vi "Database.WriteStationValues.vi"(8 "error in":errorcluster, 10 "FileName":string, 11 "Data in":T3 {"Variant"."TS"."TV"."minimum" format="%#.3f"; "Variant"."TS"."TV"."maximum" format="%#.3f"; "Variant"."TS"."TP"."value" format="%#.3f"}) -> (0 "error out":errorcluster, 3 "Data out":T3 {"Variant"."TS"."TV"."minimum" format="%#.3f"; "Variant"."TS"."TV"."maximum" format="%#.3f"; "Variant"."TS"."TP"."value" format="%#.3f"})   [LabVIEW 2016]
doc: "Write test results (measurement values) to proda database\n\nWabco 2017 All right reserved\nAuthor: maciej.szupienko@wabco-auto.com"
uses:
  Database.Main.Data.ctl
  Database.Main.Data.Status.ctl
  Database.Main.Data.Sets.ctl
  Database.Main.Data.Results.ctl
  Sequence/Sequence.Step.Status.ctl
  ProdaNG/Controls/ProdaNG.Identification.ctl
  ProdaNG/Controls/ProdaNG.ProcessResult.ctl
  ProdaNG/Controls/ProdaNG.ProcessStepResult.ctl
  ProdaNG/Controls/ProdaNG.TestStepResult.ctl
  ProdaNG/Controls/ProdaNG.TestValueResult.ctl
  Database.Main.Data.Variant.ctl
  ProdaNG/Controls/ProdaNG.ProcessStepParam.ctl
  ProdaNG/Controls/ProdaNG.TestStep.ctl
  ProdaNG/Controls/ProdaNG.TestStepParam.ctl
  ProdaNG/Controls/ProdaNG.TestValue.ctl
  tools/Translator/Translator.Message.ctl
  tools/EventLog/EventLog.EventSource.ctl
  Global/ApplicationGlobal.vi
  tools/EventLog/EventLog.New(single).vi
panel:
  out "Array 3":string[](array[string])
  out "Array 2":u64[][](array[numeric])
  out "Array":T2(array[cluster])
  out "Prod saved":bool
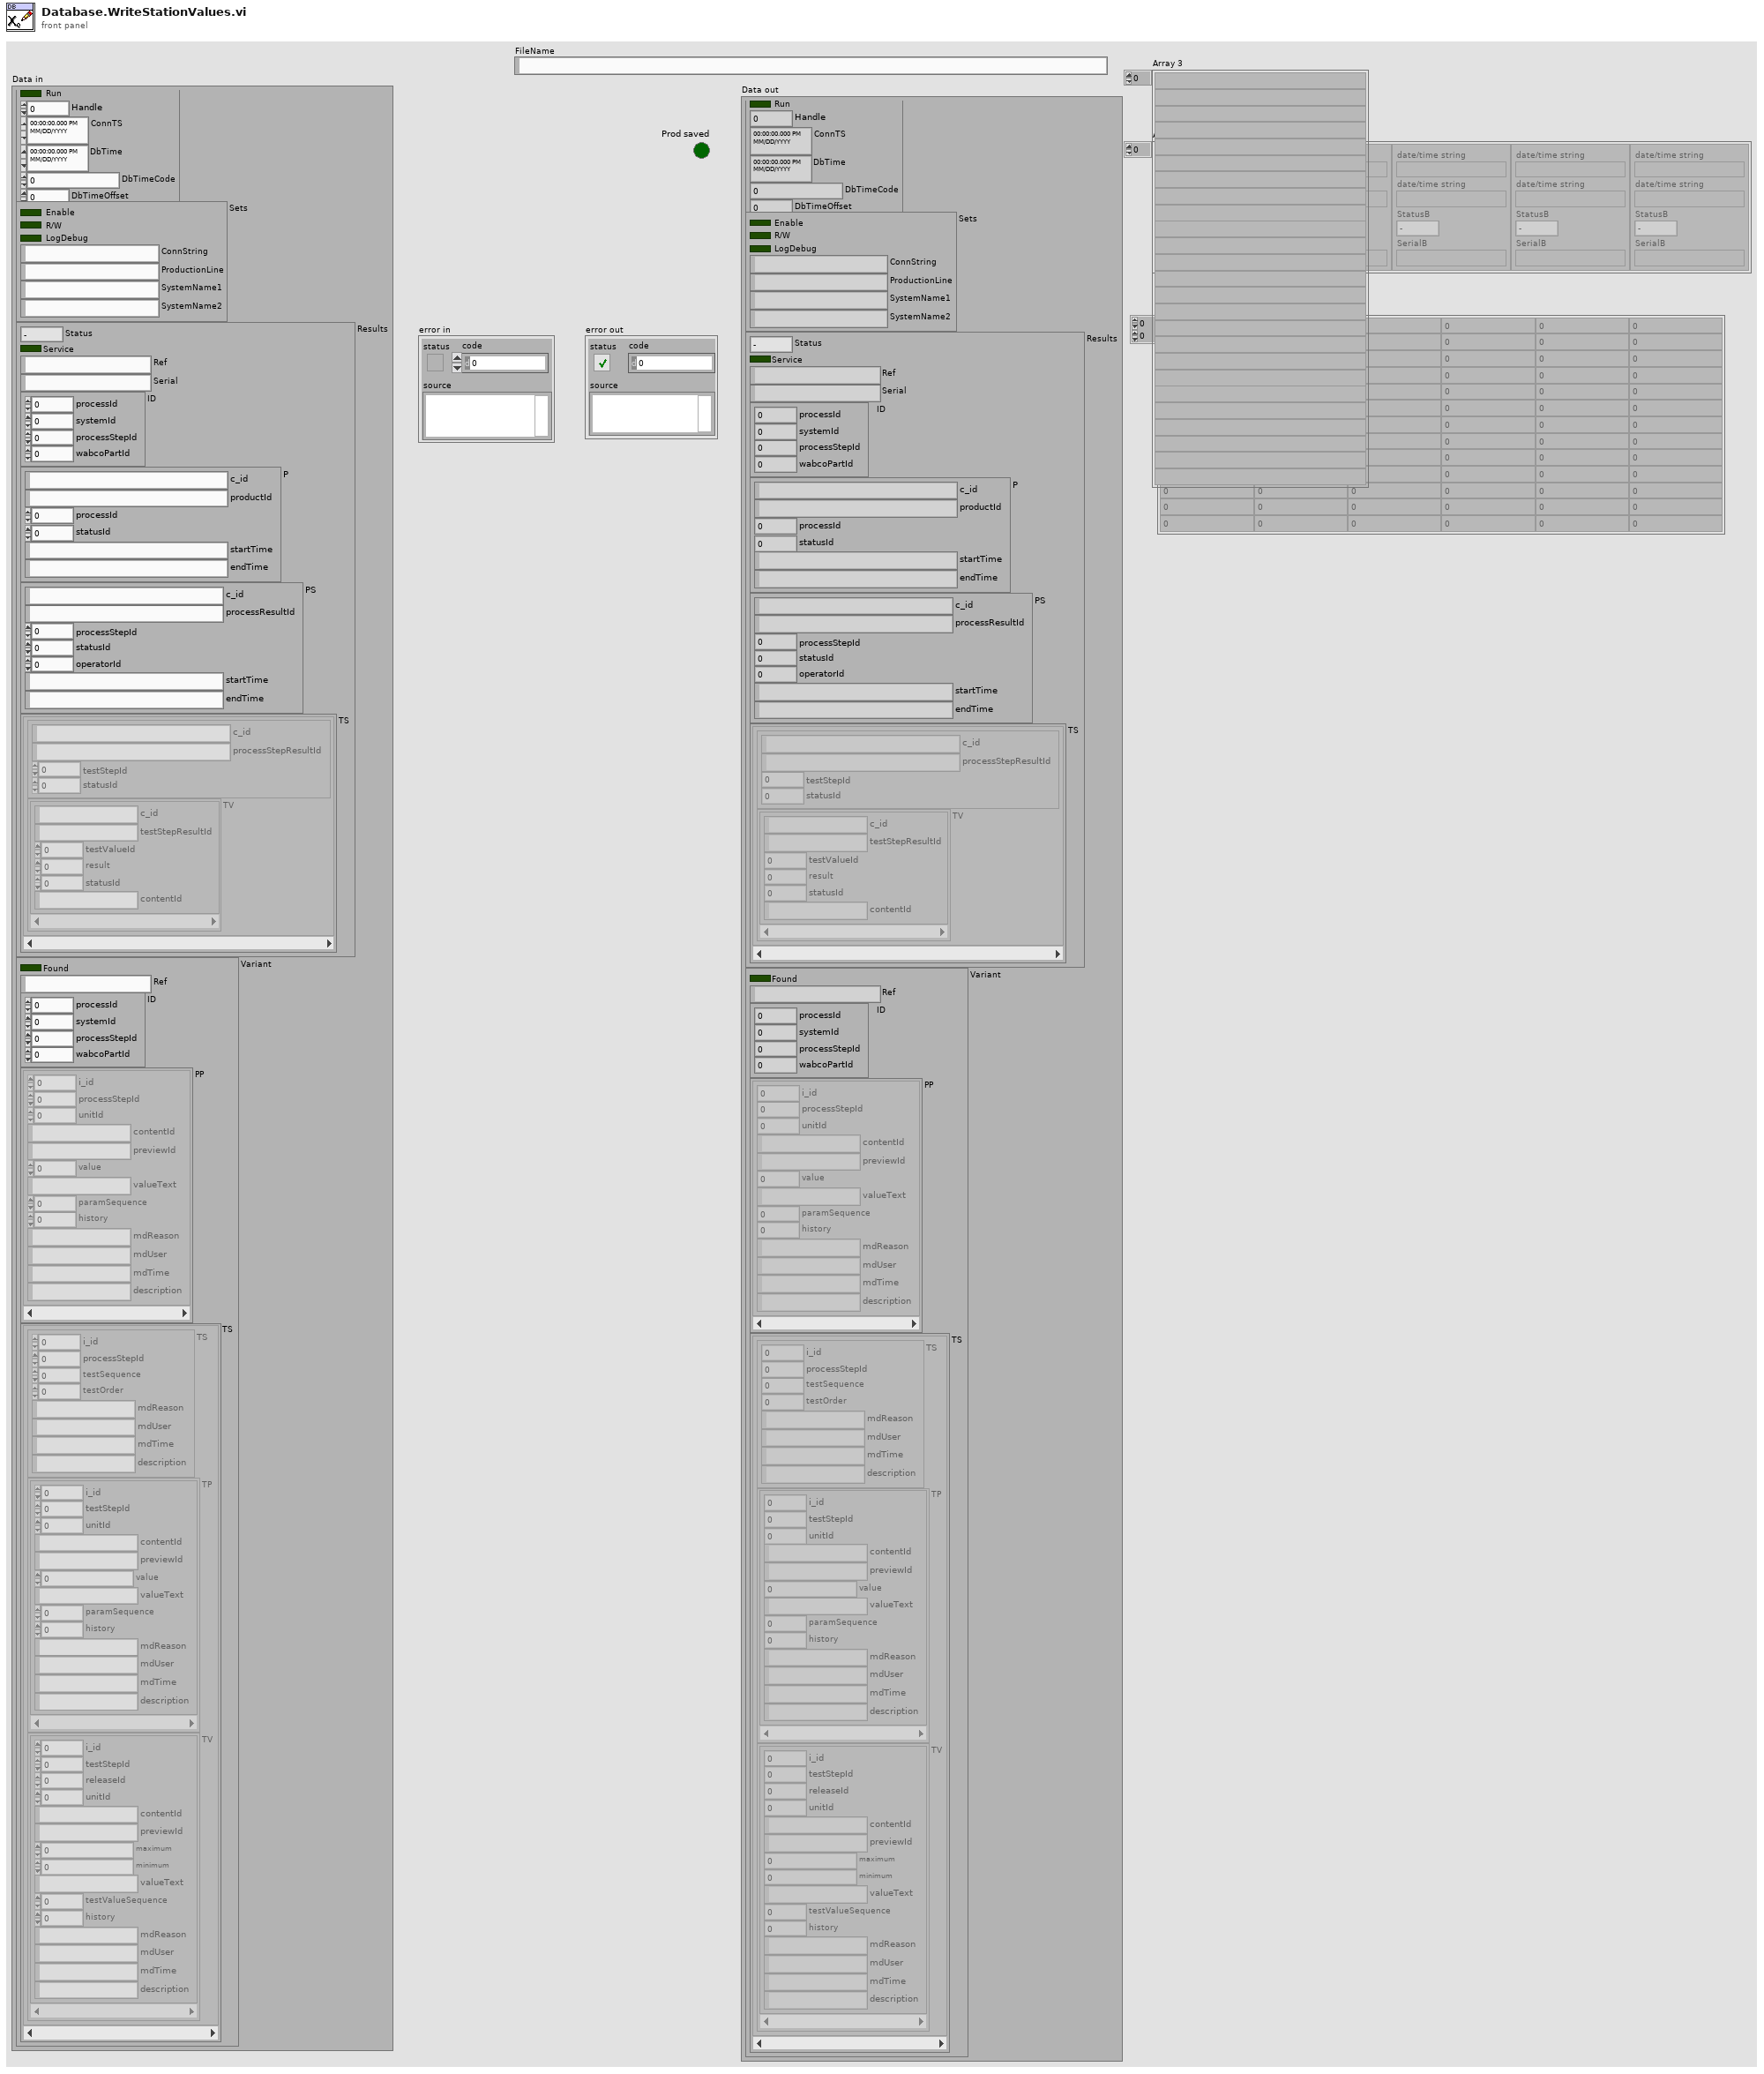
[diagram p1: front panel]
types:
  T1 = typedef "Sequence.Step.Status.ctl" = enum16{"-", "Pending", "Running", "Skipped", "Passed", "Failed", "Done", "Error", "Aborted", "Stopped"}
  T2 = cluster{"date/time string":string, "date/time string":string, "StatusB":T1, "SerialB":string}[]
  T3 = typedef "Database.Main.Data.ctl" = cluster{"Status":T4, "Sets":T5, "Results":T6, "Variant":T12}
  T4 = typedef "Database.Main.Data.Status.ctl" = cluster{"Run":bool, "Handle":i32, "ConnTS":timestamp, "DbTime":timestamp, "DbTimeCode":dbl, "DbTimeOffset":dbl}
  T5 = typedef "Database.Main.Data.Sets.ctl" = cluster{"Enable":bool, "R/W":bool, "LogDebug":bool, "ConnString":string, "ProductionLine":string, "SystemName1":string, "SystemName2":string}
  T6 = typedef "Database.Main.Data.Results.ctl" = cluster{"Status":T1, "Service":bool, "Ref":string, "Serial":string, "ID":T7, "P":T8, "PS":T9, "TS":cluster{"TS":T10, "TV":T11[]}[]}
  T7 = typedef "ProdaNG.Identification.ctl" = cluster{"processId":i32, "systemId":i32, "processStepId":i32, "wabcoPartId":i32}
  T8 = typedef "ProdaNG.ProcessResult.ctl" = cluster{"c_id":string, "productId":string, "processId":i32, "statusId":i32, "startTime":string, "endTime":string}
  T9 = typedef "ProdaNG.ProcessStepResult.ctl" = cluster{"c_id":string, "processResultId":string, "processStepId":i32, "statusId":i32, "operatorId":i32, "startTime":string, "endTime":string}
  T10 = typedef "ProdaNG.TestStepResult.ctl" = cluster{"c_id":string, "processStepResultId":string, "testStepId":i32, "statusId":i32}
  T11 = typedef "ProdaNG.TestValueResult.ctl" = cluster{"c_id":string, "testStepResultId":string, "testValueId":i32, "result":dbl, "statusId":i32, "contentId":string}
  T12 = typedef "Database.Main.Data.Variant.ctl" = cluster{"Found":bool, "Ref":string, "ID":T7, "PP":T13[], "TS":cluster{"TS":T14, "TP":T15[], "TV":T16[]}[]}
  T13 = typedef "ProdaNG.ProcessStepParam.ctl" = cluster{"i_id":i32, "processStepId":i32, "unitId":i32, "contentId":string, "previewId":string, "value":dbl, "valueText":string, "paramSequence":i32, "history":i32, "mdReason":string, "mdUser":string, "mdTime":string, "description":string}
  T14 = typedef "ProdaNG.TestStep.ctl" = cluster{"i_id":i32, "processStepId":i32, "testSequence":i32, "testOrder":i32, "mdReason":string, "mdUser":string, "mdTime":string, "description":string}
  T15 = typedef "ProdaNG.TestStepParam.ctl" = cluster{"i_id":i32, "testStepId":i32, "unitId":i32, "contentId":string, "previewId":string, "value":dbl, "valueText":string, "paramSequence":i32, "history":i32, "mdReason":string, "mdUser":string, "mdTime":string, "description":string}
  T16 = typedef "ProdaNG.TestValue.ctl" = cluster{"i_id":i32, "testStepId":i32, "releaseId":i32, "unitId":i32, "contentId":string, "previewId":string, "maximum":dbl, "minimum":dbl, "valueText":string, "testValueSequence":i32, "history":i32, "mdReason":string, "mdUser":string, "mdTime":string, "description":string}
  T17 = typedef "EventLog.EventSource.ctl" = enum16{"All", "Gui", "Ref", "File", "Arch", "Seq", "CPX", "DB", "Laser", "Scan.P", "Scan.O"}
  T18 = typedef "Translator.Message.ctl" = enum16{"-", "Event confirmed", "Log out", "Log in", "Shutdown", "Cancel", "Start", "Begin time", "End time", "Duration", "Service Mode", "Ignore Results", "Serial Format", "On", "Off", "OK", "NOK", "NOK %s", "Home", "Work", "Close", "Open", "In progress...", "Missing", "Empty", "Hardware failure", "Initial", "Default", "Total", "Out of range", "Free disk space is below 1GB - contact technician", "Error %d >> %s", "Error %d >> %s >> %s", "Msg %d >> %s", "Laser msg %d %s", "Laser cmd error %s %d", "Laser cmd failed %s", "Laser cmd warning %s", "Laser disconnected", "Laser status %s", "Laser already started", "Laser job unkonwn %s", "Laser job missing %s", "Laser job select failure %s", "Unable to start laser printing (%s)", "Unable to stop laser printing (%s)", "Laser marking aborted", "Laser marking timeout", "Unable to reset Laser Interlock (%s)", "Unable to trigger Laser. Laser not ready (%s)", "Laser job '%s' coordinates not configured", "Starting %s", "Quitting %s", "Configured", "Initializing", "Quitting", "Loading", "Loaded %d results", "Loaded %d events", "Running", "Stopped", "Summary", "Laser", "Do you want to continue?", "Do you want to delete the configuration?", "The configuration is being used by an order. Unable to delete!", "Press confirm button", "Station is not based. Do you want to exit?", "Station requires changeover. Do you want to run the test?", "Test options are not set as default. Do you want to continue?", "Formatting of WabcoNo is disabled. Do you want to continue?", "Product not detected. Do you want to continue?", "Product scan failed. Do you want to continue?", "Calibration", "Log out?", "System", "All", "IDLE", "Translating...%s", "Not found", "Alarm %s", "Run", "Skip", "Abort", "Repeat", "Please wait...", "Database disconnected", "Database disconnected - changeover disabled!", "Login to database successful", "Login to database failed: %d; %s", "Unable to check the product status of reference %d - database disconnected", "Unable to set the product status of reference %d - database disconnected", "Variant file backup %s", "Read variant (%s)", "Result", "Station armed!", "Station requires changeover!", "Select reference number...", "EMERGENCY BUTTON - press Control button", "EMERGENCY DOOR - press Control button", "Resetting Emergency...", "Unable to reset safety circuit - Emergency Button pressed", "Unable to reset safety circuit - Emergency Side Door open", "Station not based", "Station based", "Station not empty", "Station basing...", "No order", "Press Start to begin new order", "Scanning new order", "Order NOK. Correct or scan again", "Order OK. Press Accept", "Order ready", "Revolver incorrect", "Fork incorrect", "Revolver missing", "Revolver empty", "Container missing", "Offline results", "Offline statistics", "Updating statistics %.1f %%", "DMC Configurator", "Door open", "Close the front door", "Press start button", "Done. Open the front door", "Running...", "Running...%.1f %%", "Pause %s", "Pause %s. NOK container missing", "Pause %s. OK container missing", "Pause %s. Revolver empty", "Pause %s. Revolver missing", "Pause %s. Revolver incorrect", "Pause %s. Fork missing", "Pause %s. Fork incorrect", "Pause %s. Too many failures", "Pause %s. Unloading failure", "Pause %s. One slot is not working", "Pause %s. Part order is done. Empty OK container", "Pause %s. Unable to move product to slot", "Pause %s. Unable to move back product pusher", "Pause %s. Unable to lift product", "Pause %s. Unable to move back product lifter", "Pause %s. Unable to move product arm to Work", "Pause %s. Unable to move product arm to NOK", "Pause %s. Unable to move product arm to OK", "Pause %s. Unable to unsuck the NOK product", "Pause %s. Unable to drop the NOK product", "Pause %s. Product OK missing", "Pause %s. Unable to unsuck the OK product", "Pause %s. Unable to drop the OK product", "Stopping...", "File '%s' is missing", "File '%s' is broken", "File '%s' is running", "Log file started (%s)", "Log file ended (%s)", "Log file stopped (%s)", "Log file ignored (%s)", "Log file exported (%s)", "Log file export failed (%s)", "Wrong serial number in log file", "Wrong reference number in log file", "Test steps are missing", "%s = %.3f", "Process param '%s' not found in DB", "Process param '%s' wrong order", "Process param '%s' value %.3f out of limits (%.3f; %.3f)", "Step%d param '%s' not found in DB", "Step%d param '%s' wrong order", "Step%d param '%s' value %.3f out of limits (%.3f; %.3f)", "Step%d EV '%s' not found in DB", "Step%d EV '%s' wrong order", "\"%s\" not found in DB", "\"%s\" wrong order", "\"%s\" value %.3f out of limits (%.3f; %.3f)", "\"%s\" not found in software", "Process init (%s)", "Process started", "Process restarted", "Process run", "Process done", "Process done - remove OK container", "Process aborted", "Process aborted at work", "Process aborted at home", "Process error", "Process error at home", "Process error at work", "Process close", "Process pause", "Process continue", "Process door open", "Process door close", "Process pause at slot %s due to %s", "Select plate from the order to process", "Do you want to start the process?", "Do you want to continue the process?", "There is unfinished order. Do you want to put the new order?", "Product %s %d OK", "Product %s %d NOK", "Unable to unload the slot %s. Product missing in the slot", "Unable to unload the slot %s. Product already in the arm", "Unable to accept the product as OK. Product missing in slot %s", "Unable to accept the product as OK. Product could not drop into the container at slot %s", "Unable to accept the product as NOK. Product could not drop into the container at slot %s", "Scan failed. Error %s", "Scan failed. Scanner disconnected", "Scan failed. Wrong Wabco number %d, limit (%d,%d)", "Scan failed. Wrong serial number %d, limit (%d,%d)", "Scan failed. Wrong date %d, limit (%d,%d)", "Scan failed. Wrong product wabco number %d (expected %d)", "Scan failed. Wrong product serial number %d (expected > 0)", "Scan OK %s", "Scan failed. Unable to determine table position (%s)", "Scan failed. Timeout", "Tune failed. Scanner disconnected", "Tune failed. Timeout", "%s = %d", "%s = %d->%d", "Unable to set %s = %.2f - Air Pressure Inside off", "Unable to set digital output '%s' = %d", "Unable to activate air pressure inside - timeout", "Unable to activate air pressure inside - aborted", "Unable to switch on Air Main Valve - Air Pressure Inlet off", "Unable to switch on Air Main Valve - Door open", "Unable to switch off Air Main Valve - timeout", "Unable to switch off Air Main Valve - aborted", "Unable to rotate Table - timeout", "Unable to rotate Table - aborted", "Unable to rotate Table - Product Move not in Home position", "Unable to rotate Table - Air Pressure Inside off", "Unable to rotate Table - Product Lift A not in Home position", "Unable to rotate Table - Product Lift B not in Home position", "Unable to rotate Table - unlock before movement timeout", "Unable to rotate Table - lock after movement timeout", "Unable to move Table Lock to %s position - timeout", "Unable to move Table Lock to %s position - aborted", "Unable to move Table Lock to %s position - Air Pressure Inside off", "Unable to move Table Lock to %s position - Table not in position", "Unable to move Product Lift A to %s position - timeout", "Unable to move Product Lift B to %s position - timeout", "Unable to move Product Lift A to %s position - aborted", "Unable to move Product Lift B to %s position - aborted", "Unable to move Product Lift A to %s position - Air Pressure Inside off", "Unable to move Product Lift B to %s position - Air Pressure Inside off", "Unable to move Product Lift A to %s position - Table not locked", "Unable to move Product Lift B to %s position - Table not locked", "Unable to move Product Lift A to %s position - Product Arm not in Work position", "Unable to move Product Lift B to %s position - Product Arm not in Work position", "Unable to set Product Suction Gripper %s to %s - timeout", "Unable to set Product Suction Gripper %s to %s - aborted", "Unable to set Product Suction Gripper %s to %s - Air Pressure Inside off", "Unable to set Product Suction Gripper %s to %s - Table slot unkown", "Unable to move Product Arm to %s position - timeout", "Unable to move Product Arm to %s position - aborted", "Unable to move Product Arm to %s position - Air Pressure Inside off", "Unable to move Product Arm to %s position - Product Lift A not in Home position", "Unable to move Product Arm to %s position - Product Lift B not in Home position", "Unable to move Product to %s position - timeout", "Unable to move Product to %s position - aborted", "Unable to move Product to %s position - Air Pressure Inside off", "Unable to move Product to %s position - Table not in position"}
  T19 = typedef "Logger.File.ctl" = cluster{"Props":T20, "Data":T23[]}
  T20 = typedef "Logger.File.Properties.ctl" = cluster{"FilePath":path, "ImgFolder":string, "Ref":string, "Serial":string, "SerialFormat":T21, "Duration":dbl, "Time From":timestamp, "Time To":timestamp, "Service":bool, "IgnoreImgs":bool, "CheckDMC":bool, "Counters":T22, "Err":errorcluster}
  T21 = typedef "Sequence.Code.SerialFormat.ctl" = enum8{"", "6 dig", "7 dig"}
  T22 = typedef "Sequence.Counters.ctl" = cluster{"Expected":u16, "Done":u16, "OK":u16, "NOK":u16, "NOKlimit":u16, "Part":u16, "PartOK":u16}
  T23 = typedef "Logger.File.Serials.ctl" = cluster{"TS from":timestamp, "TS to":timestamp, "SlotID":u8, "StatusA":T1, "LaserVariablesA":string, "ScannerReadOutA":string, "ImgA":string, "CornersA":cluster{"X":i32, "Y":i32}[], "OCRIgnoredA":string, "SerialA":u8, "StatusB":T1, "LaserVariablesB":string, "ScannerReadOutB":string, "ImgB":string, "CornersB":cluster{"X":i32, "Y":i32}[], "SerialB":u8, "OCRIgnoredB":string, "CaptionA":string, "CaptionB":string}
  T24 = cluster{"date/time string":string, "date/time string":string, "StatusA":T1, "LaserVariablesA":string}
  T25 = cluster{"date/time string":string, "date/time string":string, "StatusB":T1, "LaserVariablesB":string}
  T26 = cluster{"date/time string":string, "date/time string":string, "StatusB":T1, "LaserVariablesB":string}[]
  T27 = typedef "ProdaNG.Product.ctl" = cluster{"c_id":string, "wabcoPartId":i32, "serialNumber":string, "comment":string, "individual":i32, "crProcessStepId":i32, "mdProcessStepId":i32, "crTime":string, "mdTime":string}
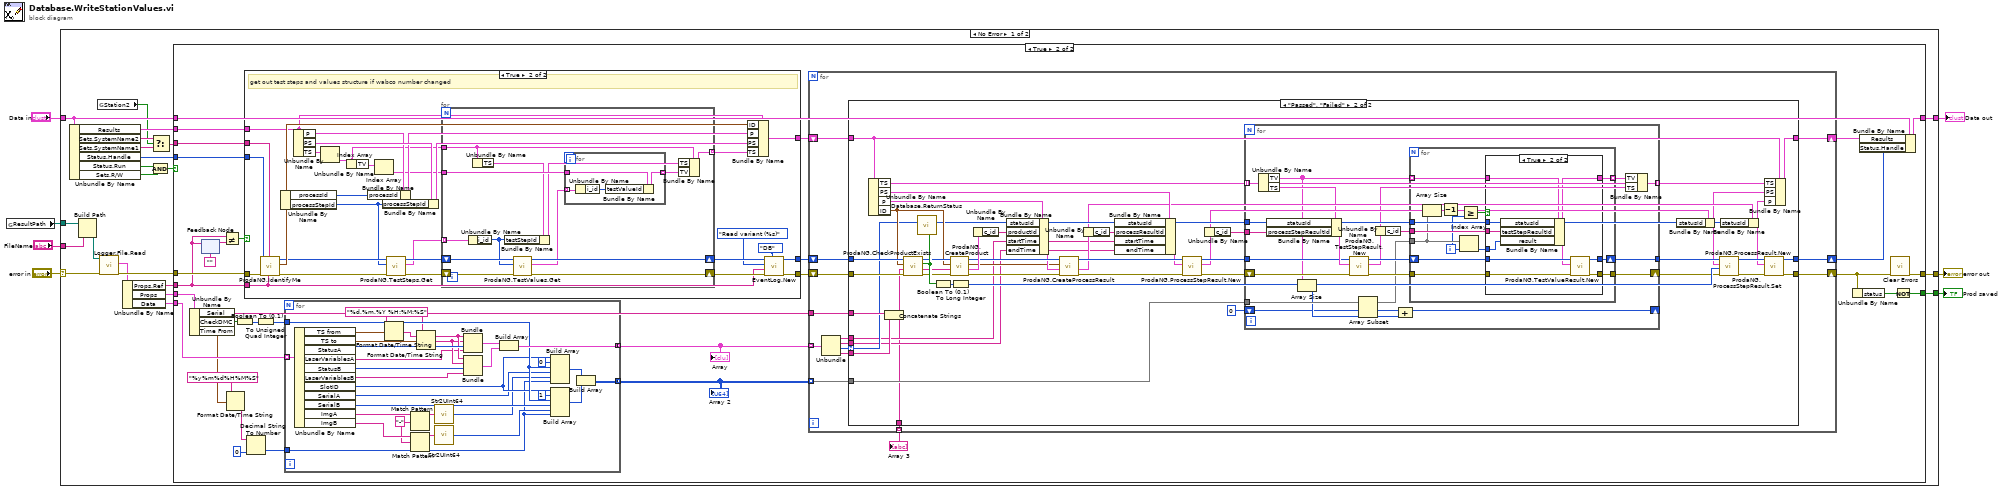
[diagram p0: block diagram]
diagram:
  n1 = global read "ApplicationGlobal.vi" "ResultPath"() -> (w2:path)
  n2 = case shown="No Error" "error in" {
    selector: "error in" -> [w13 w253]
    tunnel: [w25 w253] -> w7
    tunnel: "Data in" -> [w28 w252]
    tunnel: [w27 w252] -> w4
    tunnel: [w23 _] -> w3
    tunnel: w2 -> [w16 _]
    tunnel: "FileName" -> [w15 _]
    frame No Error {
      n3 = Unbundle By Name(w28) -> ("Results"=w26:T6, "Sets.SystemName2"=w20:string, "Sets.SystemName1"=w19:string, "Status.Handle"=w29:i32, "Status.Run"=w24:bool, "Sets.R/W"=w21:bool)
      n4 = Build Path(base path=w16, name or relative path=w15) -> (appended path=w14:path)
      n5 = global read "ApplicationGlobal.vi" "Station2"() -> (w18:bool)
      n6 = call "Logger.File.Read.vi"("error in (no error)"=w13, "file path"=w14) -> ("error out"=w12:errorcluster, "File content"=w11:T19)  [unwired: 6 in, 2 out]
      n7 = Unbundle By Name(w11) -> ("Props.Ref"=w10:string, "Props"=w8:T20, "Data"=w9:T23[])
      n8 = Select(t=w20, s=w18, f=w19) -> (s? t:f=w17:string)
      n9 = Compound Arithmetic op=AND(w24, w21) -> (w22:bool)
      n10 = case shown="True" w22 {
        tunnel: w12 -> [w31 w64]
        tunnel: w17 -> [_ w63]
        tunnel: w29 -> [_ w62]
        tunnel: w10 -> [_ w54]
        tunnel: w28 -> [w30 w61]
        tunnel: [w30 w60] -> w27
        tunnel: w26 -> [_ w59]
        tunnel: [w31 w46] -> w25
        tunnel: [_ w47] -> w23
        tunnel: w9 -> [_ w40]
        tunnel: w8 -> [_ w45]
        frame False {
        }
        frame True {
          n11 = Unbundle By Name(w45) -> ("Serial"=w44:string, "CheckDMC"=w43:bool, "Time From"=w36:timestamp)
          n12 = feedback #1("") -> (w56:string)
          n13 = feedback-in #1(w54) -> ()
          n14 = Not Equal?(x=w54, y=w56) -> (x != y?=w55:bool)
          n15 = Format Date/Time String(time format string (%c)="%y%m%d%H%M%S", seconds (now)=w36) -> (date/time string=w35:string)  [unwired: 1 in]
          n16 = Boolean To (0,1)(Boolean=w43) -> (0, 1=w42:i16)
          n17 = case shown="True" w55 {
            tunnel: w54 -> [_ w217]
            tunnel: w64 -> [w206 w224]
            tunnel: [w206 w220] -> w58
            tunnel: w63 -> [_ w222]
            tunnel: w62 -> [w205 w223]
            tunnel: [w205 w216] -> w57
            tunnel: w59 -> [w204 w214]
            tunnel: [w204 w221] -> w50
            frame False {
            }
            frame True {
              # "get out test steps and values structure if wabco number changed"
              n18 = call "ProdaNG.IdentifyMe.vi"("wabcoNumber"=w217, "systemName"=w222, "error in"=w224, "dbHandleIn"=w223) -> ("error out"=w225:errorcluster, "Identification"=w233:T7, "dbHandle"=w226:i32)  [unwired: 5 in]
              n19 = Unbundle By Name(w233) -> ("processId"=w228:i32, "processStepId"=w213:i32)
              n20 = Unbundle By Name(w214) -> ("P"=w231:T8, "PS"=w232:T9, "TS"=w211:cluster{"TS":T10, "TV":T11[]}[])
              n21 = Index Array(array=w211) -> (element=w208:cluster{"TS":T10, "TV":T11[]})  [unwired: 1 in]
              n22 = Unbundle By Name(w208) -> ("TV"=w210:T11[])
              n23 = Bundle By Name(cluster=w231, "processId"=w228) -> (w229:T8)
              n24 = Index Array(array=w210) -> (element=w209:T11)  [unwired: 1 in]
              n25 = Bundle By Name(cluster=w232, "processStepId"=w213) -> (w230:T9)
              n26 = call "ProdaNG.TestSteps.Get.vi"("error in (no error)"=w225, "processStepId"=w213, "dbHandleIn"=w226) -> ("error out"=w227:errorcluster, "TestSteps"=w212:T14[], "dbHandle"=w234:i32)  [unwired: 6 in]
              n27 = for {
                tunnel: w212 -> [w242] mode=indexing
                tunnel: w209 -> [w240]
                shift-right: [w244] -> w216
                shift-left: w234 -> [w247]
                shift-right: [w245] -> w219
                shift-left: w227 -> [w246]
                tunnel: w208 -> [w238]
                tunnel: [w235] -> w207 mode=indexing
                n28 = Unbundle By Name(w242) -> ("i_id"=w241:i32)
                n29 = Unbundle By Name(w238) -> ("TS"=w237:T10)
                n30 = Bundle By Name(cluster=w237, "testStepId"=w241) -> (w236:T10)
                n31 = call "ProdaNG.TestValues.Get.vi"("error in (no error)"=w246, "testStepId"=w241, "dbHandleIn"=w247) -> ("error out"=w245:errorcluster, "TestStepValues"=w243:T16[], "dbHandle"=w244:i32)  [unwired: 6 in]
                n32 = for {
                  tunnel: w243 -> [w251] mode=indexing
                  tunnel: w240 -> [w249]
                  tunnel: [w248] -> w239 mode=indexing
                  n33 = Unbundle By Name(w251) -> ("i_id"=w250:i32)
                  n34 = Bundle By Name(cluster=w249, "testValueId"=w250) -> (w248:T11)
                }
                n35 = Bundle By Name(cluster=w238, "TS"=w236, "TV"=w239) -> (w235:cluster{"TS":T10, "TV":T11[]})
              }
              n36 = Bundle By Name(cluster=w214, "ID"=w233, "P"=w229, "PS"=w230, "TS"=w207) -> (w221:T6)
              n37 = call-poly "EventLog.New.vi"("Source (All)"=EventLog.EventSource."DB", "error in (no error)"=w219, "Arg"=w217, "Message (-)"=Translator.Message."Read variant (%s)") -> ("error out"=w220:errorcluster)  [unwired: 6 in, 1 out]
            }
          }
          n38 = Decimal String To Number(string=w35, default (0L)=u64 0 ("default (0 I32)")) -> (number=w33:u64)  [unwired: 1 in, 1 out]
          n39 = To Unsigned Quad Integer(1:w42) -> (0:w41:u64)
          n40 = for {
            tunnel: w40 -> [w94] mode=indexing
            tunnel: [w90] -> w39 mode=concatenating
            tunnel: w41 -> [w86]
            tunnel: [w84] -> w38 mode=concatenating
            tunnel: w33 -> [w65]
            w68 = "%d.%m.%Y %H:%M:%S" ("time format string (%c)")
            w80 = "-" ("regular expression")
            n41 = Unbundle By Name(w94) -> ("TS from"=w77:timestamp, "TS to"=w76:timestamp, "StatusA"=w93:T1, "LaserVariablesA"=w67:string, "StatusB"=w92:T1, "LaserVariablesB"=w66:string, "SlotID"=w73:u8, "SerialA"=w72:u8, "SerialB"=w83:u8, "ImgA"=w71:string, "ImgB"=w81:string)
            n42 = Format Date/Time String(time format string (%c)=w68, seconds (now)=w77) -> (date/time string=w75:string)  [unwired: 1 in]
            n43 = Match Pattern(string=w71, regular expression=w80) -> (before substring=w82:string)  [unwired: 1 in, 3 out]
            n44 = Match Pattern(string=w81, regular expression=w80) -> (before substring=w79:string)  [unwired: 1 in, 3 out]
            n45 = Format Date/Time String(time format string (%c)=w68, seconds (now)=w76) -> (date/time string=w74:string)  [unwired: 1 in]
            n46 = call "Str2UInt64.vi"("string"=w82) -> ("Numeric"=w69:u64)
            n47 = call "Str2UInt64.vi"("string"=w79) -> ("Numeric"=w70:u64)
            n48 = Bundle("date/time string"=w75, "date/time string"=w74, "StatusA"=w93, "LaserVariablesA"=w67) -> (w91:T24)  [unwired: 1 in]
            n49 = Bundle("date/time string"=w75, "date/time string"=w74, "StatusB"=w92, "LaserVariablesB"=w66) -> (w89:T25)  [unwired: 1 in]
            n50 = Build Array(w91, w89) -> (w90:T26)
            n51 = Build Array(w73, u64 0, w86, w72, w69, w65) -> (w78:u64[])
            n52 = Build Array(w73, u64 1, w86, w83, w70, w65) -> (w85:u64[])
            n53 = Build Array(w78, w85) -> (w84:u64[][])
          }
          "Array" <- w39
          "Array 2" <- w38
          n54 = for {
            shift-right: [w103] -> w49
            shift-left: w58 -> [w108]
            shift-right: [w105] -> w51
            shift-left: w57 -> [w107]
            shift-right: [w106] -> w52
            shift-left: w50 -> [w104]
            tunnel: w44 -> [w101]
            tunnel: w39 -> [w102] mode=indexing
            tunnel: w38 -> [w100] mode=indexing
            tunnel: [w95] -> w32 mode=indexing
            n55 = Unbundle(w102) -> ("date/time string"=w97:string, "date/time string"=w98:string, "StatusB"=w96:T1, "LaserVariablesB"=w99:string)
            n56 = case shown="\"Passed\", \"Failed\"" w96 {
              selector: w96 -> [_ w116]
              tunnel: w108 -> [w111 w136]
              tunnel: w107 -> [w110 w135]
              tunnel: [w109 w126] -> w106
              tunnel: [w110 w122] -> w105
              tunnel: w104 -> [w109 w121]
              tunnel: [w111 w120] -> w103
              tunnel: w101 -> [_ w118]
              tunnel: w99 -> [_ w117]
              tunnel: w100 -> [_ w115]
              tunnel: w98 -> [_ w113]
              tunnel: w97 -> [_ w114]
              tunnel: [_ w112] -> w95
              frame Default {
              }
              frame "Passed", "Failed" {
                n57 = Unbundle By Name(w121) -> ("TS"=w133:cluster{"TS":T10, "TV":T11[]}[], "PS"=w132:T9, "P"=w131:T8, "ID"=w130:T7)
                n58 = Concatenate Strings(w118, w117) -> (w112:string)
                n59 = call "ProdaNG.CheckProductExists.vi"("error in (no error)"=w136, "serialNumber"=w112, "ID"=w130, "dbHandle"=w135) -> ("error out"=w138:errorcluster, "Results exist?"=w156:bool, "dbHandle out"=w134:i32)  [unwired: 2 in, 3 out]
                n60 = call "Database.ReturnStatus.vi"("repeat"=w156, "Status"=w116) -> ("Step.statusId"=w129:i32)  [unwired: 8 in, 1 out]
                n61 = Boolean To (0,1)(Boolean=w156) -> (0, 1=w137:i16)
                n62 = call "ProdaNG.CreateProduct.vi"("error in (no error)"=w138, "serialNumber"=w112, "ID"=w130, "dbHandle"=w134) -> ("error out"=w150:errorcluster, "Product out"=w155:T27, "dbHandle out"=w151:i32)  [unwired: 4 in, 1 out]
                n63 = To Long Integer(number=w137) -> (32bit integer=w154:i32)
                n64 = Unbundle By Name(w155) -> ("c_id"=w141:string)
                n65 = Bundle By Name(cluster=w131, "statusId"=w129, "productId"=w141, "startTime"=w114, "endTime"=w113) -> (w149:T8)
                n66 = call "ProdaNG.CreateProcessResult.vi"("error in (no error)"=w150, "ProcessResult"=w149, "ID"=w130, "dbHandle"=w151) -> ("error out"=w152:errorcluster, "ProcessResult 2"=w127:T8, "dbHandle out"=w153:i32)  [unwired: 5 in]
                n67 = Unbundle By Name(w127) -> ("c_id"=w142:string)
                n68 = Bundle By Name(cluster=w132, "statusId"=w129, "processResultId"=w142, "startTime"=w114, "endTime"=w113) -> (w148:T9)
                n69 = call "ProdaNG.ProcessStepResult.New.vi"("error in (no error)"=w152, "ProcessStepResult"=w148, "dbHandle"=w153) -> ("error out"=w140:errorcluster, "ProcessStepResult out"=w124:T9, "dbHandle"=w139:i32)  [unwired: 6 in]
                n70 = Unbundle By Name(w124) -> ("c_id"=w143:string)
                n71 = for {
                  tunnel: [w176] -> w145
                  tunnel: w143 -> [w174]
                  tunnel: w139 -> [w172]
                  tunnel: w115 -> [w162]
                  tunnel: w133 -> [w167] mode=indexing
                  tunnel: w129 -> [w168]
                  tunnel: [w163] -> w128 mode=indexing
                  shift-right: [w175] -> w144
                  shift-left: w140 -> [w173]
                  shift-right: [w157] -> _
                  shift-left: 0 -> [w159]
                  n72 = Unbundle By Name(w167) -> ("TV"=w161:T11[], "TS"=w165:T10)
                  n73 = Bundle By Name(cluster=w165, "statusId"=w168, "processStepResultId"=w174) -> (w177:T10)
                  n74 = Array Size(array=w161) -> (size(s)=w160:i32)
                  n75 = call "ProdaNG.TestStepResult.New.vi"("error in (no error)"=w173, "TestStepResult"=w177, "dbHandle"=w172) -> ("error out"=w169:errorcluster, "TestStepResult out"=w164:T10, "dbHandle"=w170:i32)  [unwired: 6 in]
                  n76 = Array Subset(array=w162, index=w159, length=w160) -> (w158:u64[])
                  n77 = Unbundle By Name(w164) -> ("c_id"=w171:string)
                  n78 = Compound Arithmetic op=ADD(w159, w160) -> (w157:i32)
                  n79 = for "results" {
                    tunnel: w169 -> [w191]
                    tunnel: [w188] -> w175
                    tunnel: w171 -> [w189]
                    shift-right: [w187] -> w176
                    shift-left: w170 -> [w190]
                    tunnel: w158 -> [w182]
                    tunnel: w168 -> [w186]
                    tunnel: w161 -> [w185] mode=indexing
                    tunnel: [w184] -> w166 mode=indexing
                    i -> [w180]
                    n80 = Array Size(array=w182) -> (size(s)=w179:i32)
                    n81 = Decrement(x=w179) -> (x-1=w178:i32)
                    n82 = Index Array(array=w182, index=w180) -> (element=w183:u64)
                    n83 = Greater Or Equal?(x=w178, y=w180) -> (x >= y?=w181:bool)
                    n84 = case shown="True" w181 {
                      tunnel: w191 -> [w193 w203]
                      tunnel: w190 -> [w192 w202]
                      tunnel: w189 -> [_ w201]
                      tunnel: [w193 w200] -> w188
                      tunnel: [w192 w199] -> w187
                      tunnel: w186 -> [_ w198]
                      tunnel: w185 -> [w194 w197]
                      tunnel: [w194 w196] -> w184
                      tunnel: w183 -> [_ w195]
                      frame False {
                      }
                      frame True {
                        n85 = Bundle By Name(cluster=w197, "statusId"=w198, "testStepResultId"=w201, "result"=w195) -> (w196:T11)
                        n86 = call "ProdaNG.TestValueResult.New.vi"("error in (no error)"=w203, "TestValueResult"=w196, "dbHandle"=w202) -> ("error out"=w200:errorcluster, "dbHandle"=w199:i32)  [unwired: 7 in]
                      }
                    }
                  }
                  n87 = Bundle By Name(cluster=w167, "TV"=w166, "TS"=w164) -> (w163:cluster{"TS":T10, "TV":T11[]})
                }
                n88 = Bundle By Name(cluster=w124, "statusId"=w129) -> (w123:T9)
                n89 = call "ProdaNG.ProcessStepResult.Set.vi"("error in (no error)"=w144, "isRepeat (0)"=w154, "ProcessStepResult"=w123, "dbHandle"=w145) -> ("error out"=w147:errorcluster, "dbHandle"=w146:i32)  [unwired: 6 in]
                n90 = Bundle By Name(cluster=w127, "statusId"=w129) -> (w125:T8)
                n91 = Bundle By Name(cluster=w121, "TS"=w128, "PS"=w123, "P"=w125) -> (w126:T6)
                n92 = call "ProdaNG.ProcessResult.New.vi"("error in (no error)"=w147, "ProcessResult"=w125, "dbHandle"=w146) -> ("error out"=w120:errorcluster, "dbHandle"=w122:i32)  [unwired: 6 in, 1 out]
              }
            }
          }
          "Array 3" <- w32
          n93 = Unbundle By Name(w49) -> ("status"=w48:bool)
          n94 = Bundle By Name(cluster=w61, "Results"=w52, "Status.Handle"=w51) -> (w60:T3)
          n95 = call <vilib>:"Clear Errors.vi"("error in (no error)"=w49) -> ("error out"=w46:errorcluster)  [unwired: 5 in, 1 out]
          n96 = Not(x=w48) -> (.not. x?=w47:bool)
        }
      }
    }
    frame Error {
    }
  }
  "error out" <- w7
  "Prod saved" <- w3
  "Data out" <- w4
